vi "GOOP_MyComputer_Item_Init.vi"(11 "Object":u64) -> ()   [LabVIEW 2012]
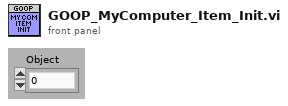
[diagram p1: front panel]
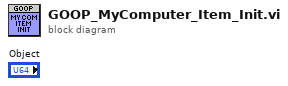
[diagram p0: block diagram]
diagram:
